vi "Is Status Null.vi"(8 "error in (no error)":errorcluster, 11 "Transfer Group Status in":refnum<class "Transfer Group Status.lvclass">) -> (0 "error out":errorcluster, 2 "null?":bool, 3 "Transfer Group Status out":refnum<class "Transfer Group Status.lvclass">)   [LabVIEW 2017, in "DSF Core.lvlib" / "Transfer Group Status.lvclass"]
uses:
  Transfer Group Status.lvclass
  C:/Program Files (x86)/National Instruments/LabVIEW 2017/vi.lib/NI/Memory Manager/Classes/Pointer/Pointer.lvclass
  <vilib>/NI/Memory Manager/Classes/Pointer/Pointer.lvclass/Pointer.ctl
  <vilib>/NI/Memory Manager/Classes/Pointer/Get Address.vi
  <vilib>/NI/Memory Manager/Classes/Pointer/Pointer.lvclass
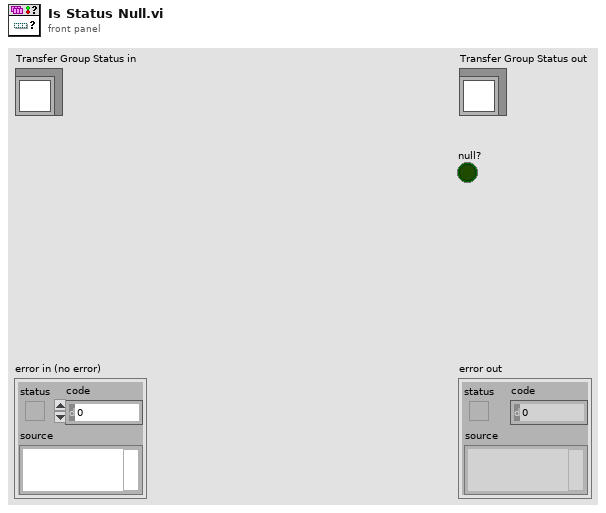
[diagram p1: front panel]
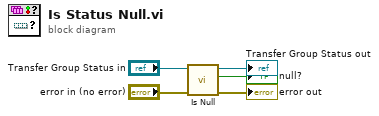
[diagram p0: block diagram]
diagram:
  n1 = call <vilib>:"Is Null.vi"("error in (no error)"="error in (no error)", "Pointer in"="Transfer Group Status in") -> ("error out"=→"error out":errorcluster, "null?"=→"null?":bool, "Pointer out"=→"Transfer Group Status out":refnum<class "Transfer Group Status.lvclass">)  [unwired: 7 in]
